vi "Read Thermo Channel.vi"(8 "error in (no error)":errorcluster, 11 "Thermo Channel configuration in":refnum<class "Thermo Channel configuration.lvclass">) -> (0 "error out":errorcluster, 2 "Thermo Channel Setting":T1={"Numeric"=0.5, "Combo"="", "String"="", "Boolean"=FALSE} {"Numeric" format="%#_f"}, 3 "Thermo Channel configuration out":refnum<class "Thermo Channel configuration.lvclass">)   [LabVIEW 2025, in "Thermo.lvlib" / "Thermo Channel configuration.lvclass"]
uses:
  Thermo Channel configuration.lvclass
  Channel Setting.ctl
  Thermo Channel configuration.lvclass/Thermo Channel configuration.ctl
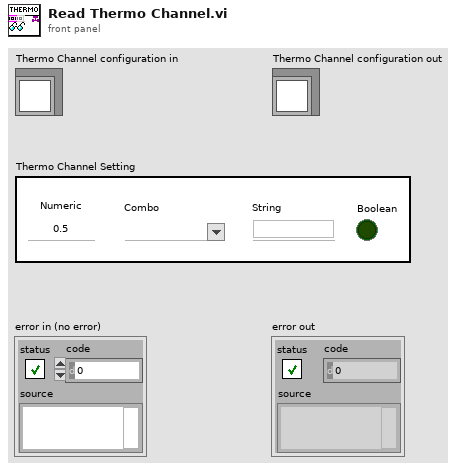
[diagram p1: front panel]
types:
  T1 = typedef "Thermo.lvlib/Thermo Channel configuration.lvclass/Channel Setting.ctl" = cluster{"Numeric":dbl, "Combo":string, "String":string, "Boolean":bool}
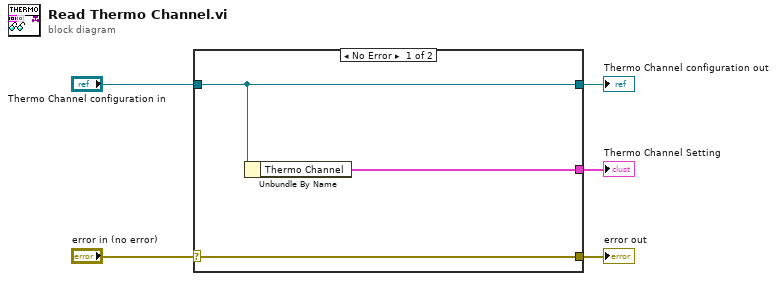
[diagram p0: block diagram]
diagram:
  n1 = case shown="No Error" "error in (no error)" {
    selector: "error in (no error)" -> [w8 w9]
    tunnel: [w8 w9] -> w4
    tunnel: [w7 w10] -> w2
    tunnel: "Thermo Channel configuration in" -> [w7 w10]
    tunnel: [w6 _] -> w1
    frame No Error {
      n2 = Unbundle By Name(w7) -> ("Thermo Channel"=w6:T1)
    }
    frame Error {
    }
  }
  "error out" <- w4
  "Thermo Channel configuration out" <- w2
  "Thermo Channel Setting" <- w1
